vi "Preview Build.vi"(8 "error in (no error)":errorcluster, 11 "Run Tests Step in":refnum<class "Run Tests Step.lvclass">) -> (0 "error out":errorcluster, 2 "Artifacts":refnum<class "Build Artifact.lvclass">[](array[class]))   [LabVIEW 2019, in "Caraya Library.lvlib" / "Run Tests Step.lvclass"]
doc: "Gets a preview of the build. This should return as much information about the artifacts as possible without actually building.\n\nDo not perform any actions that may take a long amount of time.\n\nCopyright: MGI 2016\nAuthor: Derek Trepanier"
uses:
  Run Tests Step.lvclass
  libs/Solution.lvlibp/Solution/Build Artifact/Build Artifact.lvclass
  Run Tests Step.lvclass/Run Tests Step.ctl
  libs/Project.lvlibp/Project/Binary File/Binary File.lvclass
  C:/Users/pasca/source/repos/mgi-solution-explorer-extensions/libs/Solution.lvlibp/Solution/Build Artifact/Build Artifact.lvclass
  Caraya Library.lvlib
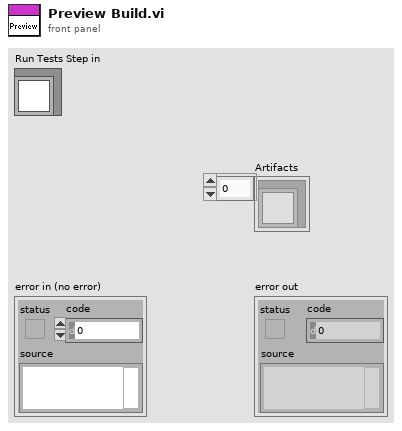
[diagram p1: front panel]
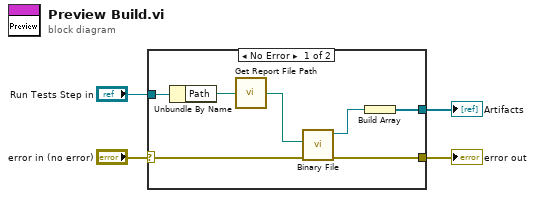
[diagram p0: block diagram]
diagram:
  n1 = case shown="No Error" "error in (no error)" {
    selector: "error in (no error)" -> [w9 w12]
    tunnel: "Run Tests Step in" -> [w11 _]
    tunnel: [w8 w12] -> w2
    tunnel: [w5 _] -> w1
    frame No Error {
      n2 = Unbundle By Name(w11) -> ("Path"=w10:path)
      n3 = call "Get Report File Path.vi"("Path"=w10) -> ("Report File"=w7:path)  [unwired: 1 in]
      n4 = call "Binary File.vi"("error in (no error)"=w9, "File"=w7) -> ("error out"=w8:errorcluster, "Binary File out"=w6:refnum<class "Binary File.lvclass">)  [unwired: 8 in]
      n5 = Build Array(w6) -> (w5:refnum<class "Binary File.lvclass">[])
    }
    frame Error {
    }
  }
  "error out" <- w2
  "Artifacts" <- w1
